vi "Dispose OCR session.vi"(8 "error in (no error)":errorcluster, 11 "IMAQ OCR Session":T1) -> (0 "error out":errorcluster)   [LabVIEW 2011]
uses:
  <vilib>/vision/OCR.llb/IMAQ OCR Session.ctl
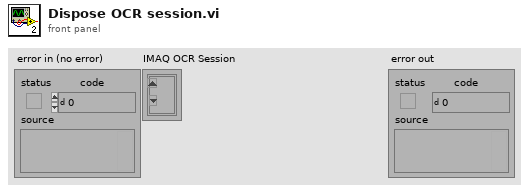
[diagram p1: front panel]
types:
  T1 = typedef "IMAQ OCR Session.ctl" = refnum<k1>
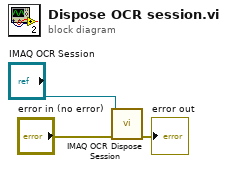
[diagram p0: block diagram]
diagram:
  n1 = call "IMAQ OCR Dispose Session"("error in (no error)"="error in (no error)", "IMAQ OCR Session"="IMAQ OCR Session") -> ("error out"=→"error out":errorcluster)  [unwired: 9 in]
